vi "Get NI-AWG Instrument Name.vi"(0 "Semiconductor Module Context":T1, 3 "error in (no error)":errorcluster) -> (7 "Semiconductor Module Context Out":T1, 8 "Instrument Names":string[](array[string]), 9 "Channel Lists":string[](array[string]), 10 "error out":errorcluster)   [LabVIEW 2013]
doc: "Returns the Channel Group Ids of all instruments of type AWG defined in the Semiconductor Module Context. You can use Instrument Names and Channel Lists to open driver sessions. The Instrument Names and Channel Lists parameters always return the same number of elements. Instrument names repeat in Instrument Names if the instrument has multiple channel groups."
uses:
  <vilib>/NI_TestStand_SemiconductorModule/NI_TestStand_Semiconductor_Module.lvlibp/PinMap/General/SemiconductorModuleContext.ctl
  <vilib>/NI_TestStand_SemiconductorModule/NI_TestStand_Semiconductor_Module.lvlibp
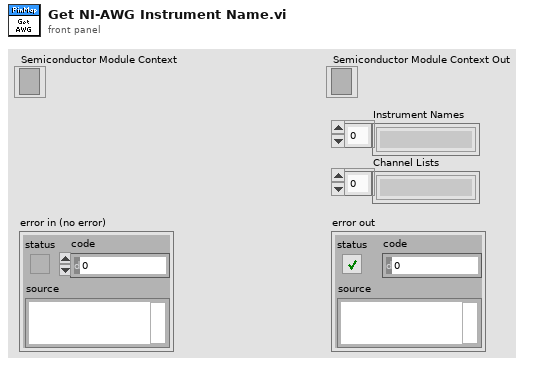
[diagram p1: front panel]
types:
  T1 = typedef "NI_TestStand_Semiconductor_Module.lvlibp/SemiconductorModuleContext.ctl" = refnum<k7>
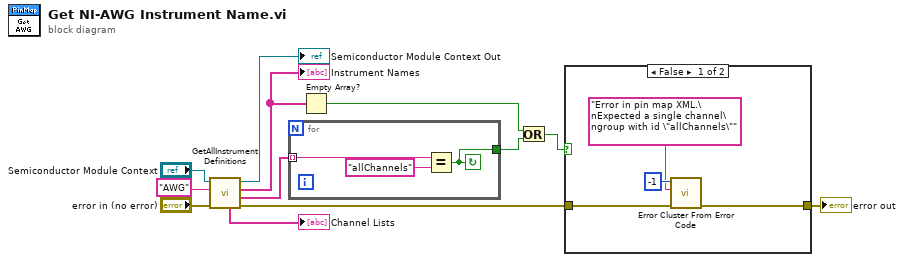
[diagram p0: block diagram]
diagram:
  n1 = call <vilib>:"GetAllInstrumentDefinitions.vi"("error in (no error)"="error in (no error)", "Instrument Type Id"="AWG", "Semiconductor Module Context"="Semiconductor Module Context") -> ("error out"=w6:errorcluster, "Channel Group Ids"=w8:string[], "Instrument Names"=w1:string[], "Semiconductor Module Context Out"=→"Semiconductor Module Context Out":T1, "Channel Lists"=→"Channel Lists":string[])  [unwired: 4 in]
  "Instrument Names" <- w1
  n2 = for {
    tunnel: w8 -> [w15] mode=indexing
    tunnel: [w13] -> w3
    stop <- w13 continue-if-true
    n3 = Equal?(x=w15, y="allChannels") -> (x = y?=w13:bool)
  }
  n4 = Empty Array?(array=w1) -> (empty?=w4:bool)
  n5 = Or(x=w4, y=w3) -> (x .or. y?=w2:bool)
  n6 = case shown="False" w2 {
    tunnel: w6 -> [w19 w20]
    tunnel: [w18 w20] -> w5
    frame False {
      n7 = call <vilib>:"Error Cluster From Error Code.vi"("error in (no error)"=w19, "error message (\"\")"="Error in pin map XML.\nExpected a single channel\ngroup with id \"allChannels\"" ("error message (\"\")"), "error code (0)"=-1) -> ("error out"=w18:errorcluster)  [unwired: 6 in]
    }
    frame True {
    }
  }
  "error out" <- w5
